vi "Draw.vi"(8 "error in (no error)":errorcluster, 10 "XY Graph":refnum<vi>, 11 "Diamond in":refnum<class "Diamond.lvclass">) -> (0 "error out":errorcluster, 3 "Diamond out":refnum<class "Diamond.lvclass">)   [LabVIEW 2023, in "d15.lvlib" / "Diamond.lvclass"]
uses:
  Diamond.lvclass
  Diamond.lvclass/Diamond.ctl
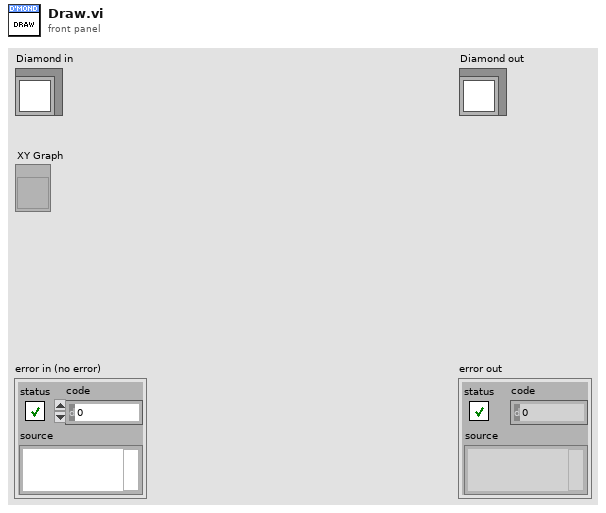
[diagram p1: front panel]
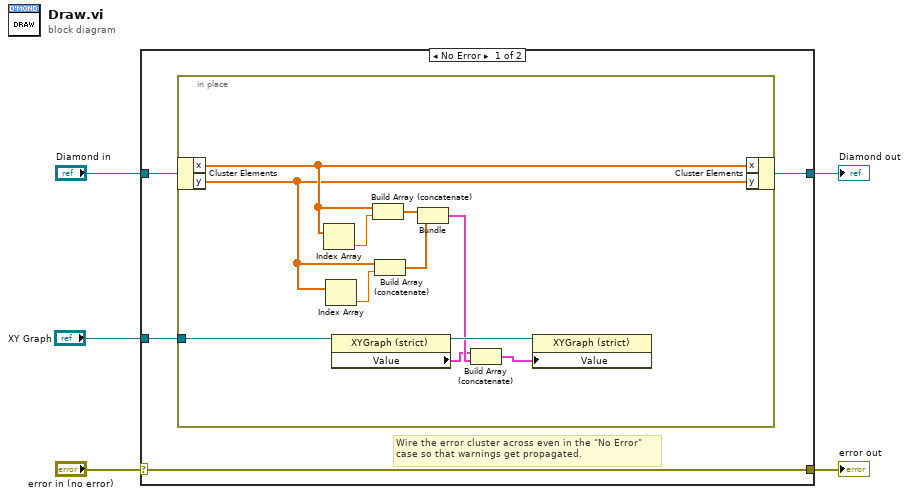
[diagram p0: block diagram]
diagram:
  n1 = case shown="No Error" "error in (no error)" {
    selector: "error in (no error)" -> [w9 w22]
    tunnel: [w9 w22] -> w4
    tunnel: [w6 w21] -> w2
    tunnel: "Diamond in" -> [w7 w21]
    tunnel: "XY Graph" -> [w8 _]
    frame No Error {
      # "Wire the error cluster across even in the \"No Error\"\ncase so that warnings get propagated."
      n2 = in-place {
        in-place-border: w8 -> [w20]
        n3 = in-place-cluster #1(w7) -> ("x"=w17:dbl[], "y"=w13:dbl[])
        n4 = Index Array(array=w17) -> (element=w15:dbl)  [unwired: 1 in]
        n5 = Index Array(array=w13) -> (element=w14:dbl)  [unwired: 1 in]
        n6 = property class="XYGraph (strict)"(reference=w20) -> (reference out=w19:refnum<vi>, "Value"=w10:cluster{"X":dbl[], "Y":dbl[]}[])  [unwired: 1 in, 1 out]
        n7 = Build Array (concatenate)(w17, w15) -> (w16:dbl[])
        n8 = Build Array (concatenate)(w13, w14) -> (w12:dbl[])
        n9 = Bundle(w16, w12) -> (w11:cluster{dbl[], dbl[]})  [unwired: 1 in]
        n10 = Build Array (concatenate)(w10, w11) -> (w18:cluster{"X":dbl[], "Y":dbl[]}[])
        n11 = property class="XYGraph (strict)"(reference=w19, "Value"=w18) -> ()  [unwired: 1 in, 2 out]
        n12 = in-place-cluster #1("x"=w17, "y"=w13) -> (w6:refnum<class "Diamond.lvclass">)
      }
    }
    frame Error {
    }
  }
  "error out" <- w4
  "Diamond out" <- w2
